vi "FindDatePath.vi"(11 "Message Value":string) -> (3 "String":string)   [LabVIEW 2013, in "main.lvlib"]
uses:
  main.lvlib
  <vilib>/regexp/Match Regular Expression.xnode
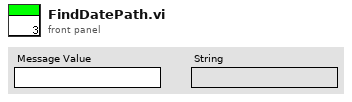
[diagram p1: front panel]
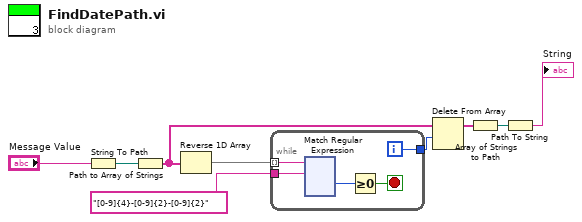
[diagram p0: block diagram]
diagram:
  n1 = String To Path(string="Message Value") -> (path=w1:path)
  n2 = Path to Array of Strings(0:w1) -> (2:w8:string[])  [unwired: 1 out]
  n3 = Reverse 1D Array(array=w8) -> (reversed array=w5:string[])
  n4 = while {
    tunnel: w5 -> [w14] mode=indexing
    tunnel: "[0-9]{4}-[0-9]{2}-[0-9]{2}" ("regular expression") -> [w12]
    tunnel: [w10] -> w4
    i -> [w10]
    stop <- w11 stop-if-true
    n5 = xnode "Match Regular Expression"("input string"=w14, "regular expression"=w12) -> ("offset past match"=w13:i32)  [unwired: 4 in, 4 out]
    n6 = Greater Or Equal To 0?(x=w13) -> (x >= 0?=w11:bool)
  }
  n7 = Delete From Array(array=w8, length=w4) -> (array with subset deleted=w9:string[])  [unwired: 1 in, 1 out]
  n8 = Array of Strings to Path(0:w9) -> (2:w6:path)  [unwired: 1 in]
  n9 = Path To String(path=w6) -> (string=→"String":string)
